vi "Main Tclk.vi"() -> ()   [LabVIEW 2018] (continued)
                                n2953 = local write "AF X tile"(w8100) -> ()
                                n2954 = local write "Auto Focus Graph"(w8101) -> ()
                                n2955 = Index Array(array=w8098, index=0) -> (element=w8097:sgl)
                                n2956 = Index Array(array=w8094, index=0) -> (element=w8093:sgl)
                              }
                              frame True {
                                n2957 = for {
                                tunnel: w8135 -> [w8165] mode=indexing
                                tunnel: w8126 -> [w8164]
                                tunnel: [w8162] -> w8127 mode=indexing
                                n2958 = for {
                                tunnel: w8165 -> [w8168] mode=indexing
                                tunnel: w8164 -> [w8167]
                                tunnel: [w8166] -> w8163 mode=indexing
                                n2959 = call "1D Parabolic Max.vi"("Y"=w8168, "X"=w8167) -> ("Xmax"=w8166:dbl)  [unwired: 2 in, 7 out]
                                }
                                n2960 = call-poly <vilib>:"Mean.vi"("X"=w8163) -> ("mean"=w8162:dbl)  [unwired: 1 out]
                                }
                                n2961 = local read "SEM Scan Parameters"() -> (w8147:T26)
                                n2962 = Initialize Array(w8143, w8152) -> (w8151:dbl[])
                                n2963 = local read "SEM Scan Parameters"() -> (w8124:T26)
                                n2964 = local read "Focus Index Options"() -> (w8112:T28)
                                n2965 = Replace Array Subset(array=w8126, new element=w8151, index=w8150) -> (w8149:sgl[])
                                n2966 = Build Cluster Array(w8126, w8155) -> (w8160:cluster{"Center":sgl, "A Img Focus Index":sgl}[])
                                n2967 = Build Cluster Array(w8153, w8154) -> (w8157:cluster{dbl, dbl}[])
                                n2968 = local write "AF Y tile"(w8109) -> ()
                                n2969 = local write "AF X tile"(w8108) -> ()
                                n2970 = Unbundle By Name(w8147) -> ("WD (mm)"=w8148:sgl[][])
                                n2971 = Unbundle By Name(w8124) -> ("X size (um)"=w8119:sgl, "X tiles"=w8118:u8, "Y size (um)"=w8116:sgl, "Y tiles"=w8115:u8)
                                n2972 = Unbundle By Name(w8112) -> ("X Grids"=w8111:u8[][], "Y Grids"=w8110:u8[][])
                                n2973 = Sort 1D Array(array=w8160) -> (sorted array=w8159:cluster{"Center":sgl, "A Img Focus Index":sgl}[])
                                n2974 = Sort 1D Array(array=w8157) -> (sorted array=w8158:cluster{dbl, dbl}[])
                                n2975 = Array Max & Min(array=w8127) -> (max value=w8132:dbl, min value=w8133:dbl)  [unwired: 2 out]
                                n2976 = Bundle(w8159) -> (w8161:T74)  [unwired: 1 in]
                                n2977 = Bundle(w8158) -> (w8156:cluster{cluster{dbl, dbl}[]})  [unwired: 1 in]
                                n2978 = Subtract(x=w8132, y=w8133) -> (x-y=w8131:dbl)
                                n2979 = Replace Array Subset(array=w8148, new element=w8143, index (row)=w8109, index (col)=w8108) -> (w8146:sgl[][])
                                n2980 = Index Array(array=w8111, index (row)=w8109, index (col)=w8108) -> (element=w8106:u8)
                                n2981 = expression code="x*0.2"(w8131) -> (w8130:dbl)
                                n2982 = Build Array(w8161, w8156) -> (w8125:T76)
                                n2983 = Divide(x=w8119, y=w8118) -> (x/y=w8117:sgl)
                                n2984 = Divide(x=w8116, y=w8115) -> (x/y=w8114:sgl)
                                n2985 = Bundle By Name(cluster=w8147, "WD (mm)"=w8146) -> (w8145:T26)
                                n2986 = local write "SEM Scan Parameters"(w8145) -> ()
                                n2987 = local write "Auto Focus Graph"(w8125) -> ()
                                n2988 = Index Array(array=w8110, index (row)=w8109, index (col)=w8108) -> (element=w8107:u8)
                                n2989 = Add(x=w8132, y=w8130) -> (x+y=w8129:dbl)
                                n2990 = Subtract(x=w8133, y=w8130) -> (x-y=w8128:dbl)
                                n2991 = call "Proportional area crop.vi"("keep aspect ratio"=w8113, "Y grids"=w8107, "Y resolution"=w8114, "X grids"=w8106, "X resolution"=w8117) -> ("Y length"=w8121:u32, "Y index"=w8122:u32[])  [unwired: 3 in, 2 out]
                                n2992 = property on="Dynamic Focus" class="XYGraph (strict)"("YScale.Maximum"=w8129, "YScale.Minimum"=w8128) -> ()  [unwired: 2 in, 2 out]
                                n2993 = expression code="x/2"(w8121) -> (w8123:u32)
                                n2994 = Add(x=w8122, y=w8123) -> (x+y=w8120:u32[])
                                n2995 = call <vilib>:"Linear Fit.vi"("Y"=w8127, "X"=w8120) -> ("Best Linear Fit"=w8137:dbl[], "slope"=w8142:dbl)  [unwired: 9 in, 3 out]
                                n2996 = expression code="x*100000"(w8142) -> (w8134:dbl)
                                n2997 = Build Cluster Array(w8120, w8127) -> (w8140:cluster{u32, "mean":dbl}[])
                                n2998 = Build Cluster Array(w8120, w8137) -> (w8141:cluster{u32, "Numeric":dbl}[])
                                n2999 = Bundle(w8140) -> (w8138:cluster{cluster{u32, "mean":dbl}[]})  [unwired: 1 in]
                                n3000 = Bundle(w8141) -> (w8139:cluster{cluster{u32, "Numeric":dbl}[]})  [unwired: 1 in]
                                n3001 = Build Array(w8138, w8139) -> (w8136:cluster{cluster{u32, "Numeric":dbl}[]}[])
                                n3002 = local write "Dynamic Focus"(w8136) -> ()
                              }
                            }
                          }
                          frame #2 {
                            n3003 = Array Size(array=w8170) -> (size(s)=w8174:i32)
                            n3004 = Greater Or Equal?(x=w8174, y=2) -> (x >= y?=w8173:bool)
                            n3005 = Array Subset(array=w8171, length=w8174) -> (w8175:sgl[])  [unwired: 1 in]
                            n3006 = case shown="True" w8173 {
                              tunnel: w8170 -> [_ w8186]
                              tunnel: w8175 -> [_ w8182]
                              tunnel: [_ w8176] -> w8169
                              frame False {
                              }
                              frame True {
                                n3007 = Array Max & Min(array=w8182) -> (max value=w8184:sgl, min value=w8183:sgl)  [unwired: 2 out]
                                n3008 = Array Max & Min(array=w8186) -> (max value=w8188:sgl, min value=w8189:sgl)  [unwired: 2 out]
                                n3009 = Subtract(x=w8184, y=w8183) -> (x-y=w8185:sgl)
                                n3010 = Subtract(x=w8188, y=w8189) -> (x-y=w8187:sgl)
                                n3011 = expression code="x*0.2"(w8185) -> (w8181:sgl)
                                n3012 = expression code="x*0.2"(w8187) -> (w8190:sgl)
                                n3013 = Add(x=w8184, y=w8181) -> (x+y=w8180:sgl)
                                n3014 = Subtract(x=w8183, y=w8181) -> (x-y=w8179:sgl)
                                n3015 = Add(x=w8188, y=w8190) -> (x+y=w8178:sgl)
                                n3016 = Subtract(x=w8189, y=w8190) -> (x-y=w8177:sgl)
                                n3017 = property on="Auto Focus Graph" class="XYGraph (strict)"("XScale.Maximum"=w8180, "XScale.Minimum"=w8179, "YScale.Maximum"=w8178, "YScale.Minimum"=w8177) -> ()  [unwired: 2 in, 2 out]
                                n3018 = Bundle(w8180, w8179, w8178, w8177) -> (w8176:cluster{sgl, sgl, sgl, sgl})  [unwired: 1 in]
                              }
                            }
                          }
                        }
                      }
                    }
                    n3019 = local write "Auto Focus Graph tiled"(w7977) -> ()
                    n3020 = local write "Best WD (mm) tiled"(w7984) -> ()
                    n3021 = local write "AF Graph scales tiled"(w7976) -> ()
                    n3022 = local write "WD array tiled"(w7987) -> ()
                    n3023 = local write "AF Success tiled"(w7983) -> ()
                    n3024 = local write "Best WD FI tiled"(w7985) -> ()
                    n3025 = local write "Skip Steps tiled"(w7986) -> ()
                    n3026 = local write "Slope tiled"(w7979) -> ()
                    n3027 = And Array Elements(Boolean array=w7981) -> (logical AND=w7978:bool)
                    n3028 = case shown="True" w7978 {
                      frame False {
                      }
                      frame True {
                        w7995 = T44."Enabled" ("Disabled")
                        w7997 = sgl[][][] [] ("FI array tiled")
                        n3029 = local write "Auto Focus"(FALSE ("Rect Milling Line Paused")) -> ()
                        n3030 = local write "AF Count"(u8 0 ("AF Count")) -> ()
                        n3031 = local write "Skip Steps tiled"(u8[][] [] ("AS Count tiled")) -> ()
                        n3032 = local write "FI array tiled"(w7997) -> ()
                        n3033 = local write "WD array tiled"(w7997) -> ()
                        n3034 = local write "FI grid array tiled"(sgl[][][][][] [] ("FI grid array tiled")) -> ()
                        n3035 = property on="Auto Align" class="Bool (strict)"("DisabledEnum"=w7995) -> ()  [unwired: 2 in, 2 out]
                        n3036 = property on="Auto Stig" class="Bool (strict)"("DisabledEnum"=w7995) -> ()  [unwired: 2 in, 2 out]
                        n3037 = property on="Auto Focus" class="Bool (strict)"("DisabledEnum"=w7995) -> ()  [unwired: 2 in, 2 out]
                        n3038 = property on="AF Steps" class="DigNum (strict)"("DisabledEnum"=w7995) -> ()  [unwired: 2 in, 2 out]
                        n3039 = property on="Keep aspect ratio" class="Bool (strict)"("DisabledEnum"=w7995) -> ()  [unwired: 2 in, 2 out]
                        n3040 = property on="X Grids" class="Arr (strict)"("DisabledEnum"=w7995) -> ()  [unwired: 2 in, 2 out]
                        n3041 = property on="Y Grids" class="Arr (strict)"("DisabledEnum"=w7995) -> ()  [unwired: 2 in, 2 out]
                        n3042 = property on="Primary X index" class="Arr (strict)"("DisabledEnum"=w7995) -> ()  [unwired: 2 in, 2 out]
                        n3043 = property on="Primary Y index" class="Arr (strict)"("DisabledEnum"=w7995) -> ()  [unwired: 2 in, 2 out]
                      }
                    }
                  }
                  frame True {
                  }
                }
              }
              frame #32 {
                n3044 = local read "StigX array tiled"() -> (w8192:sgl[][][])
                n3045 = local read "FI array tiled"() -> (w8193:sgl[][][])
                n3046 = local read "AS Count"() -> (w8194:u8)
                n3047 = local read "AS Steps"() -> (w8196:u8)
                n3048 = local read "Skip Steps tiled"() -> (w8195:u8[][])
                n3049 = local read "Auto Stig"() -> (w8197:bool)
                n3050 = Empty Array?(array=w8192) -> (empty?=w8191:bool)
                n3051 = Not(x=w8197) -> (.not. x?=w8198:bool)
                n3052 = case shown="False" w8191 {
                  tunnel: w8192 -> [w8213 _]
                  tunnel: w8193 -> [w8212 _]
                  tunnel: w8194 -> [w8211 _]
                  tunnel: w8195 -> [w8210 _]
                  tunnel: w8196 -> [w8209 _]
                  tunnel: w8198 -> [w8203 _]
                  frame False {
                    n3053 = for {
                      tunnel: w8213 -> [w8237] mode=indexing
                      tunnel: w8212 -> [w8236] mode=indexing
                      tunnel: w8211 -> [w8235]
                      tunnel: w8210 -> [w8234] mode=indexing
                      tunnel: w8209 -> [w8233]
                      tunnel: [w8232] -> w8208 mode=indexing
                      tunnel: [w8230] -> w8207 mode=indexing
                      tunnel: [w8229] -> w8206 mode=indexing
                      tunnel: [w8228] -> w8205 mode=indexing
                      tunnel: [w8227] -> w8204 mode=indexing
                      tunnel: w8203 -> [w8226]
                      tunnel: [w8225] -> w8202 mode=indexing
                      tunnel: [w8224] -> w8200 mode=indexing
                      tunnel: [w8223] -> w8199 mode=indexing
                      i -> [w8231]
                      n3054 = for {
                        tunnel: w8237 -> [w8253] mode=indexing
                        tunnel: w8236 -> [w8252] mode=indexing
                        tunnel: w8235 -> [w8251]
                        tunnel: w8234 -> [w8250] mode=indexing
                        tunnel: w8233 -> [w8249]
                        tunnel: [w8248] -> w8232 mode=indexing
                        tunnel: w8231 -> [w8247]
                        tunnel: [w8245] -> w8230 mode=indexing
                        tunnel: [w8244] -> w8229 mode=indexing
                        tunnel: [w8243] -> w8228 mode=indexing
                        tunnel: [w8242] -> w8227 mode=indexing
                        tunnel: w8226 -> [w8241]
                        tunnel: [w8240] -> w8225 mode=indexing
                        tunnel: [w8239] -> w8224 mode=indexing
                        tunnel: [w8238] -> w8223 mode=indexing
                        i -> [w8246]
                        n3055 = stacked-sequence {
                          seq-local: [w8256 _ _] -> [_ w8294 _]
                          seq-local: [w8254 _ _] -> [_ w8285 _]
                          tunnel: w8253 -> [w8261 w8286 w8341]
                          tunnel: w8252 -> [w8260 w8299 w8340]
                          tunnel: w8251 -> [w8258 w8282 _]
                          tunnel: w8250 -> [w8255 _ _]
                          tunnel: w8249 -> [w8257 w8283 _]
                          tunnel: [_ w8295 _] -> w8248
                          tunnel: w8247 -> [_ w8293 _]
                          tunnel: w8246 -> [_ w8292 _]
                          tunnel: [w8254 _ _] -> w8245
                          tunnel: [_ w8291 _] -> w8244
                          tunnel: [_ w8290 _] -> w8243
                          tunnel: [_ w8289 _] -> w8242
                          tunnel: w8241 -> [_ w8288 _]
                          tunnel: [_ w8287 _] -> w8240
                          tunnel: [_ _ w8339] -> w8239
                          tunnel: [_ w8284 _] -> w8238
                          frame #0 {
                            n3056 = Subtract(x=w8257, y=w8255) -> (x-y=w8259:u8)
                            n3057 = Less?(x=w8258, y=w8259) -> (x < y?=w8262:bool)
                            n3058 = case shown="True" w8262 {
                              tunnel: w8261 -> [w8264 w8269]
                              tunnel: w8258 -> [_ w8268]
                              tunnel: w8260 -> [_ w8270]
                              tunnel: [w8264 w8267] -> w8256
                              tunnel: w8255 -> [w8263 w8266]
                              tunnel: [w8263 w8265] -> w8254
                              frame False {
                              }
                              frame True {
                                n3059 = Index Array(array=w8269, index=w8268) -> (element=w8272:sgl)
                                n3060 = call "1D Parabolic Max.vi"("Y"=w8270, "Xt"=w8272, "X"=w8269) -> ("Y(Xt) < Ymin"=w8271:bool)  [unwired: 1 in, 7 out]
                                n3061 = case shown="True" w8271 {
                                tunnel: w8268 -> [_ w8278]
                                tunnel: w8269 -> [w8274 w8279]
                                tunnel: w8266 -> [w8273 w8276]
                                tunnel: [w8274 w8277] -> w8267
                                tunnel: [w8273 w8275] -> w8265
                                frame False {
                                }
                                frame True {
                                n3062 = Delete From Array(array=w8279, length=1, index=w8278) -> (array with subset deleted=w8277:sgl[])  [unwired: 1 out]
                                n3063 = Increment(x=w8276) -> (x+1=w8275:u8)
                                }
                                }
                              }
                            }
                          }
                          frame #1 {
                            n3064 = Subtract(x=w8283, y=w8285) -> (x-y=w8298:u8)
                            n3065 = call "1D Parabolic Max.vi"("Y"=w8299, "X"=w8286) -> ("Found max"=w8289:bool, "Ymax"=w8296:dbl, "Xmax"=w8300:dbl, "Finer Best Polynomial Fit"=w8302:dbl[], "Finer X"=w8297:dbl[])  [unwired: 2 in, 3 out]
                            n3066 = Greater Or Equal?(x=w8282, y=w8298) -> (x >= y?=w8301:bool)
                            n3067 = Subtract(x=w8283, y=w8282) -> (x-y=w8281:u8)
                            n3068 = Compound Arithmetic op=OR(w8289, w8301, w8288) -> (w8287:bool)
                            n3069 = case shown="True" w8287 {
                              tunnel: w8300 -> [_ w8320]
                              tunnel: w8299 -> [w8304 w8332]
                              tunnel: w8294 -> [w8312 _]
                              tunnel: w8302 -> [_ w8331]
                              tunnel: w8297 -> [_ w8330]
                              tunnel: w8296 -> [_ w8321]
                              tunnel: w8281 -> [_ w8329]
                              tunnel: w8282 -> [_ w8327]
                              tunnel: [w8312 w8326] -> w8295
                              tunnel: w8293 -> [w8309 w8318]
                              tunnel: w8292 -> [w8310 w8317]
                              tunnel: [w8303 w8321] -> w8291
                              tunnel: [w8306 w8320] -> w8290
                              tunnel: w8286 -> [w8308 w8319]
                              tunnel: [w8311 w8316] -> w8284
                              frame False {
                                n3070 = Build Cluster Array(w8308, w8304) -> (w8313:cluster{"Center":sgl, "A Img Focus Index":sgl}[])
                                n3071 = Sort 1D Array(array=w8313) -> (sorted array=w8314:cluster{"Center":sgl, "A Img Focus Index":sgl}[])
                                n3072 = Bundle(w8314) -> (w8315:T74)  [unwired: 1 in]
                                n3073 = Build Array(w8315) -> (w8311:T75)
                                n3074 = local write "ASX Y tile"(w8309) -> ()
                                n3075 = local write "ASX X tile"(w8310) -> ()
                                n3076 = local write "Auto Stig X"(w8311) -> ()
                                n3077 = Index Array(array=w8308, index=0) -> (element=w8306:sgl)
                                n3078 = Index Array(array=w8304, index=0) -> (element=w8303:sgl)
                              }
                              frame True {
                                n3079 = local read "SEM Scan Parameters"() -> (w8324:T26)
                                n3080 = Initialize Array(w8320, w8329) -> (w8328:dbl[])
                                n3081 = Replace Array Subset(array=w8319, new element=w8328, index=w8327) -> (w8326:sgl[])
                                n3082 = Unbundle By Name(w8324) -> ("X stig"=w8325:sgl[][])
                                n3083 = Build Cluster Array(w8319, w8332) -> (w8337:cluster{"Center":sgl, "A Img Focus Index":sgl}[])
                                n3084 = Build Cluster Array(w8330, w8331) -> (w8334:cluster{dbl, dbl}[])
                                n3085 = local write "ASX Y tile"(w8318) -> ()
                                n3086 = local write "ASX X tile"(w8317) -> ()
                                n3087 = Sort 1D Array(array=w8337) -> (sorted array=w8336:cluster{"Center":sgl, "A Img Focus Index":sgl}[])
                                n3088 = Sort 1D Array(array=w8334) -> (sorted array=w8335:cluster{dbl, dbl}[])
                                n3089 = Replace Array Subset(array=w8325, new element=w8320, index (row)=w8318, index (col)=w8317) -> (w8323:sgl[][])
                                n3090 = Bundle(w8336) -> (w8338:T74)  [unwired: 1 in]
                                n3091 = Bundle(w8335) -> (w8333:cluster{cluster{dbl, dbl}[]})  [unwired: 1 in]
                                n3092 = Bundle By Name(cluster=w8324, "X stig"=w8323) -> (w8322:T26)
                                n3093 = local write "SEM Scan Parameters"(w8322) -> ()
                                n3094 = Build Array(w8338, w8333) -> (w8316:T76)
                                n3095 = local write "Auto Stig X"(w8316) -> ()
                              }
                            }
                          }
                          frame #2 {
                            n3096 = Array Size(array=w8340) -> (size(s)=w8343:i32)
                            n3097 = Greater Or Equal?(x=w8343, y=2) -> (x >= y?=w8344:bool)
                            n3098 = Array Subset(array=w8341, length=w8343) -> (w8342:sgl[])  [unwired: 1 in]
                            n3099 = case shown="True" w8344 {
                              tunnel: w8340 -> [_ w8356]
                              tunnel: w8342 -> [_ w8352]
                              tunnel: [_ w8346] -> w8339
                              frame False {
                              }
                              frame True {
                                n3100 = Array Max & Min(array=w8352) -> (max value=w8354:sgl, min value=w8353:sgl)  [unwired: 2 out]
                                n3101 = Array Max & Min(array=w8356) -> (max value=w8358:sgl, min value=w8359:sgl)  [unwired: 2 out]
                                n3102 = Subtract(x=w8354, y=w8353) -> (x-y=w8355:sgl)
                                n3103 = Subtract(x=w8358, y=w8359) -> (x-y=w8357:sgl)
                                n3104 = expression code="x*0.2"(w8355) -> (w8351:sgl)
                                n3105 = expression code="x*0.2"(w8357) -> (w8360:sgl)
                                n3106 = Add(x=w8354, y=w8351) -> (x+y=w8350:sgl)
                                n3107 = Subtract(x=w8353, y=w8351) -> (x-y=w8349:sgl)
                                n3108 = Add(x=w8358, y=w8360) -> (x+y=w8348:sgl)
                                n3109 = Subtract(x=w8359, y=w8360) -> (x-y=w8347:sgl)
                                n3110 = Bundle(w8350, w8349, w8348, w8347) -> (w8346:cluster{sgl, sgl, sgl, sgl})  [unwired: 1 in]
                                n3111 = property on="Auto Stig X" class="XYGraph (strict)"("XScale.Maximum"=w8350, "XScale.Minimum"=w8349, "YScale.Maximum"=w8348, "YScale.Minimum"=w8347) -> ()  [unwired: 2 in, 2 out]
                              }
                            }
                          }
                        }
                      }
                    }
                    n3112 = And Array Elements(Boolean array=w8202) -> (logical AND=w8201:bool)
                    n3113 = local write "ASX Success tiled"(w8204) -> ()
                    n3114 = local write "Best Stig X (%) tiled"(w8205) -> ()
                    n3115 = local write "ASX Graph scales tiled"(w8200) -> ()
                    n3116 = local write "StigX array tiled"(w8208) -> ()
                    n3117 = local write "ASX Graph tiled"(w8199) -> ()
                    n3118 = local write "Best Stig X FI tiled"(w8206) -> ()
                    n3119 = local write "Skip Steps tiled"(w8207) -> ()
                    n3120 = case shown="True" w8201 {
                      frame False {
                      }
                      frame True {
                        w8220 = sgl[][][] [] ("FI array tiled")
                        w8222 = T44."Enabled" ("Disabled")
                        n3121 = local read "SEM Scan Parameters"() -> (w8219:T26)
                        n3122 = Unbundle By Name(w8219) -> ("Y tiles"=w8215:u8, "X tiles"=w8216:u8)
                        n3123 = local write "AS Count"(u8 0 ("AS Count")) -> ()
                        n3124 = local write "FI array tiled"(w8220) -> ()
                        n3125 = local write "StigX array tiled"(w8220) -> ()
                        n3126 = local write "Stig Options"(enum16{"Defaut", "Stig X", "Stig Y"}."Stig Y" ("Stig Options")) -> ()
                        n3127 = property on="Auto Stig" class="Bool (strict)"("DisabledEnum"=w8222) -> ()  [unwired: 2 in, 2 out]
                        n3128 = property on="AS Steps" class="DigNum (strict)"("DisabledEnum"=w8222) -> ()  [unwired: 2 in, 2 out]
                        n3129 = Initialize Array(u8 0 ("Skip Steps"), w8215, w8216) -> (w8217:u8[][])
                        n3130 = local write "Skip Steps tiled"(w8217) -> ()
                      }
                    }
                  }
                  frame True {
                  }
                }
              }
              frame #33 {
                n3131 = local read "StigY array tiled"() -> (w8362:sgl[][][])
                n3132 = local read "FI array tiled"() -> (w8363:sgl[][][])
                n3133 = local read "AS Count"() -> (w8364:u8)
                n3134 = local read "AS Steps"() -> (w8366:u8)
                n3135 = local read "Skip Steps tiled"() -> (w8365:u8[][])
                n3136 = local read "Auto Stig"() -> (w8367:bool)
                n3137 = Empty Array?(array=w8362) -> (empty?=w8361:bool)
                n3138 = Not(x=w8367) -> (.not. x?=w8368:bool)
                n3139 = case shown="False" w8361 {
                  tunnel: w8362 -> [w8383 _]
                  tunnel: w8363 -> [w8382 _]
                  tunnel: w8364 -> [w8381 _]
                  tunnel: w8365 -> [w8380 _]
                  tunnel: w8366 -> [w8379 _]
                  tunnel: w8368 -> [w8373 _]
                  frame False {
                    n3140 = for {
                      tunnel: w8383 -> [w8404] mode=indexing
                      tunnel: w8382 -> [w8403] mode=indexing
                      tunnel: w8381 -> [w8402]
                      tunnel: w8380 -> [w8401] mode=indexing
                      tunnel: w8379 -> [w8400]
                      tunnel: [w8399] -> w8378 mode=indexing
                      tunnel: [w8397] -> w8377 mode=indexing
                      tunnel: [w8396] -> w8376 mode=indexing
                      tunnel: [w8395] -> w8375 mode=indexing
                      tunnel: [w8394] -> w8374 mode=indexing
                      tunnel: w8373 -> [w8393]
                      tunnel: [w8392] -> w8372 mode=indexing
                      tunnel: [w8391] -> w8370 mode=indexing
                      tunnel: [w8390] -> w8369 mode=indexing
                      i -> [w8398]
                      n3141 = for {
                        tunnel: w8404 -> [w8420] mode=indexing
                        tunnel: w8403 -> [w8419] mode=indexing
                        tunnel: w8402 -> [w8418]
                        tunnel: w8401 -> [w8417] mode=indexing
                        tunnel: w8400 -> [w8416]
                        tunnel: [w8415] -> w8399 mode=indexing
                        tunnel: w8398 -> [w8414]
                        tunnel: [w8412] -> w8397 mode=indexing
                        tunnel: [w8411] -> w8396 mode=indexing
                        tunnel: [w8410] -> w8395 mode=indexing
                        tunnel: [w8409] -> w8394 mode=indexing
                        tunnel: w8393 -> [w8408]
                        tunnel: [w8407] -> w8392 mode=indexing
                        tunnel: [w8406] -> w8391 mode=indexing
                        tunnel: [w8405] -> w8390 mode=indexing
                        i -> [w8413]
                        n3142 = stacked-sequence {
                          seq-local: [w8423 _ _] -> [_ w8461 _]
                          seq-local: [w8421 _ _] -> [_ w8452 _]
                          tunnel: w8420 -> [w8428 w8453 w8508]
                          tunnel: w8419 -> [w8427 w8466 w8507]
                          tunnel: w8418 -> [w8425 w8449 _]
                          tunnel: w8417 -> [w8422 _ _]
                          tunnel: w8416 -> [w8424 w8450 _]
                          tunnel: [_ w8462 _] -> w8415
                          tunnel: w8414 -> [_ w8460 _]
                          tunnel: w8413 -> [_ w8459 _]
                          tunnel: [w8421 _ _] -> w8412
                          tunnel: [_ w8458 _] -> w8411
                          tunnel: [_ w8457 _] -> w8410
                          tunnel: [_ w8456 _] -> w8409
                          tunnel: w8408 -> [_ w8455 _]
                          tunnel: [_ w8454 _] -> w8407
                          tunnel: [_ w8451 _] -> w8406
                          tunnel: [_ _ w8506] -> w8405
                          frame #0 {
                            n3143 = Subtract(x=w8424, y=w8422) -> (x-y=w8426:u8)
                            n3144 = Less?(x=w8425, y=w8426) -> (x < y?=w8429:bool)
                            n3145 = case shown="True" w8429 {
                              tunnel: w8428 -> [w8431 w8436]
                              tunnel: w8425 -> [_ w8435]
                              tunnel: w8427 -> [_ w8437]
                              tunnel: [w8431 w8434] -> w8423
                              tunnel: w8422 -> [w8430 w8433]
                              tunnel: [w8430 w8432] -> w8421
                              frame False {
                              }
                              frame True {
                                n3146 = Index Array(array=w8436, index=w8435) -> (element=w8439:sgl)
                                n3147 = call "1D Parabolic Max.vi"("Y"=w8437, "Xt"=w8439, "X"=w8436) -> ("Y(Xt) < Ymin"=w8438:bool)  [unwired: 1 in, 7 out]
                                n3148 = case shown="False" w8438 {
                                tunnel: w8435 -> [_ w8445]
                                tunnel: w8436 -> [w8441 w8446]
                                tunnel: w8433 -> [w8440 w8443]
                                tunnel: [w8441 w8444] -> w8434
                                tunnel: [w8440 w8442] -> w8432
                                frame False {
                                }
                                frame True {
                                n3149 = Delete From Array(array=w8446, length=1, index=w8445) -> (array with subset deleted=w8444:sgl[])  [unwired: 1 out]
                                n3150 = Increment(x=w8443) -> (x+1=w8442:u8)
                                }
                                }
                              }
                            }
                          }
                          frame #1 {
                            n3151 = Subtract(x=w8450, y=w8452) -> (x-y=w8465:u8)
                            n3152 = call "1D Parabolic Max.vi"("Y"=w8466, "X"=w8453) -> ("Found max"=w8456:bool, "Ymax"=w8463:dbl, "Xmax"=w8467:dbl, "Finer Best Polynomial Fit"=w8469:dbl[], "Finer X"=w8464:dbl[])  [unwired: 2 in, 3 out]
                            n3153 = Greater Or Equal?(x=w8449, y=w8465) -> (x >= y?=w8468:bool)
                            n3154 = Subtract(x=w8450, y=w8449) -> (x-y=w8448:u8)
                            n3155 = Compound Arithmetic op=OR(w8456, w8468, w8455) -> (w8454:bool)
                            n3156 = case shown="True" w8454 {
                              tunnel: w8467 -> [_ w8487]
                              tunnel: w8466 -> [w8471 w8499]
                              tunnel: w8461 -> [w8479 _]
                              tunnel: w8469 -> [_ w8498]
                              tunnel: w8464 -> [_ w8497]
                              tunnel: w8463 -> [_ w8488]
                              tunnel: w8448 -> [_ w8496]
                              tunnel: w8449 -> [_ w8494]
                              tunnel: [w8479 w8493] -> w8462
                              tunnel: w8460 -> [w8476 w8484]
                              tunnel: w8459 -> [w8477 w8483]
                              tunnel: [w8470 w8488] -> w8458
                              tunnel: [w8473 w8487] -> w8457
                              tunnel: w8453 -> [w8475 w8486]
                              tunnel: [w8478 w8485] -> w8451
                              frame False {
                                n3157 = Build Cluster Array(w8475, w8471) -> (w8480:cluster{"Center":sgl, "A Img Focus Index":sgl}[])
                                n3158 = Sort 1D Array(array=w8480) -> (sorted array=w8481:cluster{"Center":sgl, "A Img Focus Index":sgl}[])
                                n3159 = Bundle(w8481) -> (w8482:T74)  [unwired: 1 in]
                                n3160 = Build Array(w8482) -> (w8478:T75)
                                n3161 = local write "ASY Y tile"(w8476) -> ()
                                n3162 = local write "ASY X tile"(w8477) -> ()
                                n3163 = local write "Auto Stig Y"(w8478) -> ()
                                n3164 = Index Array(array=w8475, index=0) -> (element=w8473:sgl)
                                n3165 = Index Array(array=w8471, index=0) -> (element=w8470:sgl)
                              }
                              frame True {
                                n3166 = local read "SEM Scan Parameters"() -> (w8491:T26)
                                n3167 = Initialize Array(w8487, w8496) -> (w8495:dbl[])
                                n3168 = Replace Array Subset(array=w8486, new element=w8495, index=w8494) -> (w8493:sgl[])
                                n3169 = Unbundle By Name(w8491) -> ("Y stig"=w8492:sgl[][])
                                n3170 = Build Cluster Array(w8486, w8499) -> (w8504:cluster{"Center":sgl, "A Img Focus Index":sgl}[])
                                n3171 = Build Cluster Array(w8497, w8498) -> (w8501:cluster{dbl, dbl}[])
                                n3172 = local write "ASY Y tile"(w8484) -> ()
                                n3173 = local write "ASY X tile"(w8483) -> ()
                                n3174 = Sort 1D Array(array=w8504) -> (sorted array=w8503:cluster{"Center":sgl, "A Img Focus Index":sgl}[])
                                n3175 = Sort 1D Array(array=w8501) -> (sorted array=w8502:cluster{dbl, dbl}[])
                                n3176 = Replace Array Subset(array=w8492, new element=w8487, index (row)=w8484, index (col)=w8483) -> (w8490:sgl[][])
                                n3177 = Bundle(w8503) -> (w8505:T74)  [unwired: 1 in]
                                n3178 = Bundle(w8502) -> (w8500:cluster{cluster{dbl, dbl}[]})  [unwired: 1 in]
                                n3179 = Bundle By Name(cluster=w8491, "Y stig"=w8490) -> (w8489:T26)
                                n3180 = local write "SEM Scan Parameters"(w8489) -> ()
                                n3181 = Build Array(w8505, w8500) -> (w8485:T76)
                                n3182 = local write "Auto Stig Y"(w8485) -> ()
                              }
                            }
                          }
                          frame #2 {
                            n3183 = Array Size(array=w8507) -> (size(s)=w8509:i32)
                            n3184 = Greater Or Equal?(x=w8509, y=2) -> (x >= y?=w8511:bool)
                            n3185 = Array Subset(array=w8508, length=w8509) -> (w8510:sgl[])  [unwired: 1 in]
                            n3186 = case shown="True" w8511 {
                              tunnel: w8507 -> [_ w8523]
                              tunnel: w8510 -> [_ w8519]
                              tunnel: [_ w8513] -> w8506
                              frame False {
                              }
                              frame True {
                                n3187 = Array Max & Min(array=w8519) -> (max value=w8521:sgl, min value=w8520:sgl)  [unwired: 2 out]
                                n3188 = Array Max & Min(array=w8523) -> (max value=w8525:sgl, min value=w8526:sgl)  [unwired: 2 out]
                                n3189 = Subtract(x=w8521, y=w8520) -> (x-y=w8522:sgl)
                                n3190 = Subtract(x=w8525, y=w8526) -> (x-y=w8524:sgl)
                                n3191 = expression code="x*0.2"(w8522) -> (w8518:sgl)
                                n3192 = expression code="x*0.2"(w8524) -> (w8527:sgl)
                                n3193 = Add(x=w8521, y=w8518) -> (x+y=w8517:sgl)
                                n3194 = Subtract(x=w8520, y=w8518) -> (x-y=w8516:sgl)
                                n3195 = Add(x=w8525, y=w8527) -> (x+y=w8515:sgl)
                                n3196 = Subtract(x=w8526, y=w8527) -> (x-y=w8514:sgl)
                                n3197 = Bundle(w8517, w8516, w8515, w8514) -> (w8513:cluster{sgl, sgl, sgl, sgl})  [unwired: 1 in]
                                n3198 = property on="Auto Stig Y" class="XYGraph (strict)"("XScale.Maximum"=w8517, "XScale.Minimum"=w8516, "YScale.Maximum"=w8515, "YScale.Minimum"=w8514) -> ()  [unwired: 2 in, 2 out]
                              }
                            }
                          }
                        }
                      }
                    }
                    n3199 = And Array Elements(Boolean array=w8372) -> (logical AND=w8371:bool)
                    n3200 = local write "ASY Success tiled"(w8374) -> ()
                    n3201 = local write "Best Stig Y (%) tiled"(w8375) -> ()
                    n3202 = local write "ASY Graph scales tiled"(w8369) -> ()
                    n3203 = local write "StigY array tiled"(w8378) -> ()
                    n3204 = local write "ASY Graph tiled"(w8370) -> ()
                    n3205 = local write "Best Stig Y FI tiled"(w8376) -> ()
                    n3206 = local write "Skip Steps tiled"(w8377) -> ()
                    n3207 = case shown="True" w8371 {
                      frame False {
                      }
                      frame True {
                        w8386 = T44."Enabled" ("Disabled")
                        w8387 = sgl[][][] [] ("FI array tiled")
                        n3208 = local write "Auto Stig"(FALSE ("Auto Stig")) -> ()
                        n3209 = local write "AS Count"(u8 0 ("AS Count")) -> ()
                        n3210 = local write "Skip Steps tiled"(u8[][] [] ("AS Count tiled")) -> ()
                        n3211 = local write "FI array tiled"(w8387) -> ()
                        n3212 = local write "StigY array tiled"(w8387) -> ()
                        n3213 = local write "Stig Options"(enum16{"Defaut", "Stig X", "Stig Y"}."Defaut" ("Stig Options")) -> ()
                        n3214 = property on="Auto Focus" class="Bool (strict)"("DisabledEnum"=w8386) -> ()  [unwired: 2 in, 2 out]
                        n3215 = property on="Auto Stig" class="Bool (strict)"("DisabledEnum"=w8386) -> ()  [unwired: 2 in, 2 out]
                        n3216 = property on="Auto Align" class="Bool (strict)"("DisabledEnum"=w8386) -> ()  [unwired: 2 in, 2 out]
                        n3217 = property on="AS Steps" class="DigNum (strict)"("DisabledEnum"=w8386) -> ()  [unwired: 2 in, 2 out]
                      }
                    }
                  }
                  frame True {
                  }
                }
              }
              frame #34 {
                n3218 = local read "AlnX array tiled"() -> (w8529:sgl[][][])
                n3219 = local read "FI array tiled"() -> (w8530:sgl[][][])
                n3220 = local read "AA Count"() -> (w8531:u8)
                n3221 = local read "AA Steps"() -> (w8533:u8)
                n3222 = local read "Skip Steps tiled"() -> (w8532:u8[][])
                n3223 = local read "Auto Align"() -> (w8534:bool)
                n3224 = Empty Array?(array=w8529) -> (empty?=w8528:bool)
                n3225 = Not(x=w8534) -> (.not. x?=w8535:bool)
                n3226 = case shown="False" w8528 {
                  tunnel: w8529 -> [w8550 _]
                  tunnel: w8530 -> [w8549 _]
                  tunnel: w8531 -> [w8548 _]
                  tunnel: w8532 -> [w8547 _]
                  tunnel: w8533 -> [w8546 _]
                  tunnel: w8535 -> [w8540 _]
                  frame False {
                    n3227 = for {
                      tunnel: w8550 -> [w8574] mode=indexing
                      tunnel: w8549 -> [w8573] mode=indexing
                      tunnel: w8548 -> [w8572]
                      tunnel: w8547 -> [w8571] mode=indexing
                      tunnel: w8546 -> [w8570]
                      tunnel: [w8569] -> w8545 mode=indexing
                      tunnel: [w8567] -> w8544 mode=indexing
                      tunnel: [w8566] -> w8543 mode=indexing
                      tunnel: [w8565] -> w8542 mode=indexing
                      tunnel: [w8564] -> w8541 mode=indexing
                      tunnel: w8540 -> [w8563]
                      tunnel: [w8562] -> w8539 mode=indexing
                      tunnel: [w8561] -> w8537 mode=indexing
                      tunnel: [w8560] -> w8536 mode=indexing
                      i -> [w8568]
                      n3228 = for {
                        tunnel: w8574 -> [w8590] mode=indexing
                        tunnel: w8573 -> [w8589] mode=indexing
                        tunnel: w8572 -> [w8588]
                        tunnel: w8571 -> [w8587] mode=indexing
                        tunnel: w8570 -> [w8586]
                        tunnel: [w8585] -> w8569 mode=indexing
                        tunnel: w8568 -> [w8584]
                        tunnel: [w8582] -> w8567 mode=indexing
                        tunnel: [w8581] -> w8566 mode=indexing
                        tunnel: [w8580] -> w8565 mode=indexing
                        tunnel: [w8579] -> w8564 mode=indexing
                        tunnel: w8563 -> [w8578]
                        tunnel: [w8577] -> w8562 mode=indexing
                        tunnel: [w8576] -> w8561 mode=indexing
                        tunnel: [w8575] -> w8560 mode=indexing
                        i -> [w8583]
                        n3229 = stacked-sequence {
                          seq-local: [w8593 _ _] -> [_ w8631 _]
                          seq-local: [w8591 _ _] -> [_ w8622 _]
                          tunnel: w8590 -> [w8598 w8623 w8678]
                          tunnel: w8589 -> [w8597 w8636 w8677]
                          tunnel: w8588 -> [w8595 w8619 _]
                          tunnel: w8587 -> [w8592 _ _]
                          tunnel: w8586 -> [w8594 w8620 _]
                          tunnel: [_ w8632 _] -> w8585
                          tunnel: w8584 -> [_ w8630 _]
                          tunnel: w8583 -> [_ w8629 _]
                          tunnel: [w8591 _ _] -> w8582
                          tunnel: [_ w8628 _] -> w8581
                          tunnel: [_ w8627 _] -> w8580
                          tunnel: [_ w8626 _] -> w8579
                          tunnel: w8578 -> [_ w8625 _]
                          tunnel: [_ w8624 _] -> w8577
                          tunnel: [_ w8621 _] -> w8576
                          tunnel: [_ _ w8676] -> w8575
                          frame #0 {
                            n3230 = Subtract(x=w8594, y=w8592) -> (x-y=w8596:u8)
                            n3231 = Less?(x=w8595, y=w8596) -> (x < y?=w8599:bool)
                            n3232 = case shown="True" w8599 {
                              tunnel: w8598 -> [w8601 w8606]
                              tunnel: w8595 -> [_ w8605]
                              tunnel: w8597 -> [_ w8607]
                              tunnel: [w8601 w8604] -> w8593
                              tunnel: w8592 -> [w8600 w8603]
                              tunnel: [w8600 w8602] -> w8591
                              frame False {
                              }
                              frame True {
                                n3233 = Index Array(array=w8606, index=w8605) -> (element=w8609:sgl)
                                n3234 = call "1D Parabolic Max.vi"("Y"=w8607, "Xt"=w8609, "X"=w8606) -> ("Y(Xt) < Ymin"=w8608:bool)  [unwired: 1 in, 7 out]
                                n3235 = case shown="False" w8608 {
                                tunnel: w8605 -> [_ w8615]
                                tunnel: w8606 -> [w8611 w8616]
                                tunnel: w8603 -> [w8610 w8613]
                                tunnel: [w8611 w8614] -> w8604
                                tunnel: [w8610 w8612] -> w8602
                                frame False {
                                }
                                frame True {
                                n3236 = Delete From Array(array=w8616, length=1, index=w8615) -> (array with subset deleted=w8614:sgl[])  [unwired: 1 out]
                                n3237 = Increment(x=w8613) -> (x+1=w8612:u8)
                                }
                                }
                              }
                            }
                          }
                          frame #1 {
                            n3238 = Subtract(x=w8620, y=w8622) -> (x-y=w8635:u8)
                            n3239 = call "1D Parabolic Max.vi"("Y"=w8636, "X"=w8623) -> ("Found max"=w8626:bool, "Ymax"=w8633:dbl, "Xmax"=w8637:dbl, "Finer Best Polynomial Fit"=w8639:dbl[], "Finer X"=w8634:dbl[])  [unwired: 2 in, 3 out]
                            n3240 = Greater Or Equal?(x=w8619, y=w8635) -> (x >= y?=w8638:bool)
                            n3241 = Subtract(x=w8620, y=w8619) -> (x-y=w8618:u8)
                            n3242 = Compound Arithmetic op=OR(w8626, w8638, w8625) -> (w8624:bool)
                            n3243 = case shown="True" w8624 {
                              tunnel: w8637 -> [_ w8657]
                              tunnel: w8636 -> [w8641 w8669]
                              tunnel: w8631 -> [w8649 _]
                              tunnel: w8639 -> [_ w8668]
                              tunnel: w8634 -> [_ w8667]
                              tunnel: w8633 -> [_ w8658]
                              tunnel: w8618 -> [_ w8666]
                              tunnel: w8619 -> [_ w8664]
                              tunnel: [w8649 w8663] -> w8632
                              tunnel: w8630 -> [w8646 w8654]
                              tunnel: w8629 -> [w8647 w8653]
                              tunnel: [w8640 w8658] -> w8628
                              tunnel: [w8644 w8657] -> w8627
                              tunnel: w8623 -> [w8645 w8656]
                              tunnel: [w8648 w8655] -> w8621
                              frame False {
                                n3244 = Build Cluster Array(w8645, w8641) -> (w8650:cluster{"Center":sgl, "A Img Focus Index":sgl}[])
                                n3245 = Sort 1D Array(array=w8650) -> (sorted array=w8651:cluster{"Center":sgl, "A Img Focus Index":sgl}[])
                                n3246 = Bundle(w8651) -> (w8652:T74)  [unwired: 1 in]
                                n3247 = Build Array(w8652) -> (w8648:T75)
                                n3248 = local write "AAX Y tile"(w8646) -> ()
                                n3249 = local write "AAX X tile"(w8647) -> ()
                                n3250 = local write "Auto Aln X"(w8648) -> ()
                                n3251 = Index Array(array=w8645, index=0) -> (element=w8644:sgl)
                                n3252 = Index Array(array=w8641, index=0) -> (element=w8640:sgl)
                              }
                              frame True {
                                n3253 = local read "SEM Scan Parameters"() -> (w8661:T26)
                                n3254 = Initialize Array(w8657, w8666) -> (w8665:dbl[])
                                n3255 = Replace Array Subset(array=w8656, new element=w8665, index=w8664) -> (w8663:sgl[])
                                n3256 = Build Cluster Array(w8656, w8669) -> (w8674:cluster{"Center":sgl, "A Img Focus Index":sgl}[])
                                n3257 = Build Cluster Array(w8667, w8668) -> (w8671:cluster{dbl, dbl}[])
                                n3258 = local write "AAX Y tile"(w8654) -> ()
                                n3259 = local write "AAX X tile"(w8653) -> ()
                                n3260 = Unbundle By Name(w8661) -> ("X aln"=w8662:sgl[][])
                                n3261 = Sort 1D Array(array=w8674) -> (sorted array=w8673:cluster{"Center":sgl, "A Img Focus Index":sgl}[])
                                n3262 = Sort 1D Array(array=w8671) -> (sorted array=w8672:cluster{dbl, dbl}[])
                                n3263 = Replace Array Subset(array=w8662, new element=w8657, index (row)=w8654, index (col)=w8653) -> (w8660:sgl[][])
                                n3264 = Bundle(w8673) -> (w8675:T74)  [unwired: 1 in]
                                n3265 = Bundle(w8672) -> (w8670:cluster{cluster{dbl, dbl}[]})  [unwired: 1 in]
                                n3266 = Bundle By Name(cluster=w8661, "X aln"=w8660) -> (w8659:T26)
